vi "Create UserEventHandler.vi"(8 "error in":errorcluster, 9 "Name":string, 10 "Level":T1) -> (0 "error out":errorcluster, 3 "UserEventHandler out":refnum<class "UserEventHandler.lvclass">)   [LabVIEW 2020, in "hse-logger.lvlib" / "UserEventHandler.lvclass"]
doc: "Creates and initializes a new UserEventHandler object.\n\n____\nHAMPEL SOFTWARE ENGINEERING v2.0.6 (2021-04-15 11:38)"
uses:
  UserEventHandler.lvclass
  LogLevel.ctl
  hse-logger.lvlib
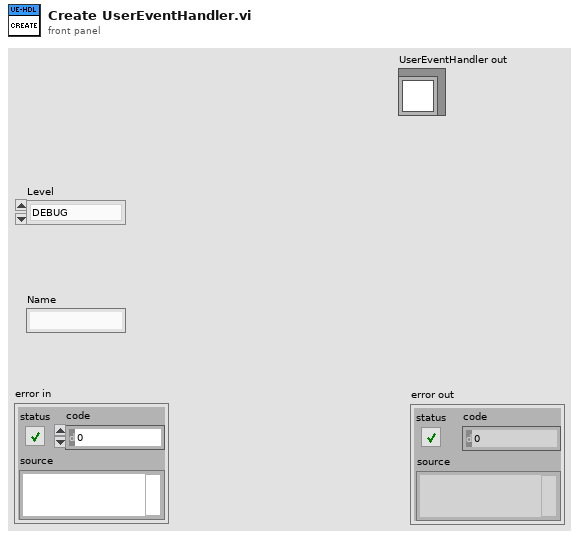
[diagram p1: front panel]
types:
  T1 = typedef "hse-logger.lvlib/LogLevel.ctl" = enum16{"DEBUG", "INFO", "WARNING", "ERROR", "CRITICAL"}
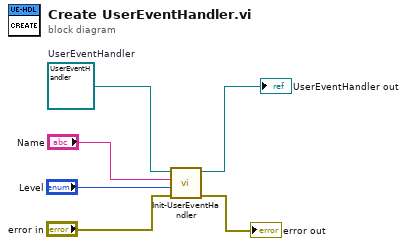
[diagram p0: block diagram]
diagram:
  w3 = refnum<class "UserEventHandler.lvclass"> refnum  # UserEventHandler
  n1 = call-dynamic "Init-UserEventHandler.vi"("error in"="error in", "Level"="Level", "Name"="Name", "UserEventHandler"=w3) -> ("error out"=→"error out":errorcluster, "UserEventHandler out"=→"UserEventHandler out":refnum<class "UserEventHandler.lvclass">)  [unwired: 6 in]
